vi "NewPeriodic Tasks.vi"(8 "error in":errorcluster) -> ()   [LabVIEW 2017]
doc: "This VI runs in parallel to other tasks. It can contain as many user-defined periodic loops as you need. These can carry out PID or other sorts of timed response."
uses:
  <vilib>/Analysis/baseanly.llb/Mean (DBL).vi
  <vilib>/Rock Robotics/WPI/Utilities/WPI_GetSetVariantRefNum.vi
  Robot Global Data.vi
  <vilib>/Rock Robotics/Network Tables/NT Write Number.vi
  <vilib>/Rock Robotics/Network Tables/NT Write Numeric Array.vi
  <vilib>/Analysis/NI_AALBase.lvlib
panel:
  out "Arrayval":dbl
  out "Accelerations":T1
  out "Joy Y":dbl(graph)
  out "Avg Y":dbl
  out "Mean":dbl(graph)
  out "Current Joy Y Value":dbl
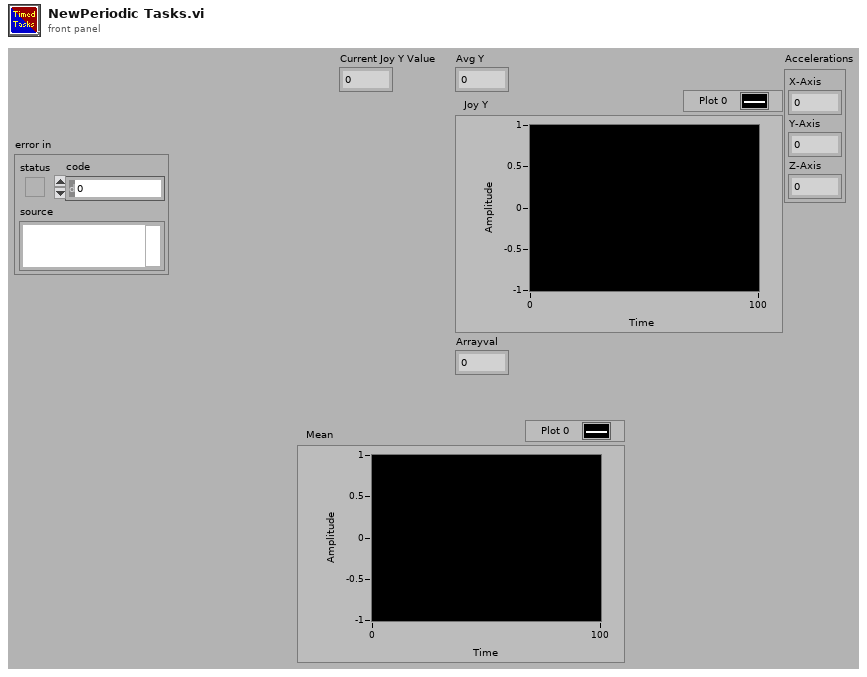
[diagram p1: front panel]
types:
  T1 = cluster{"X-Axis":dbl, "Y-Axis":dbl, "Z-Axis":dbl}
  T2 = typedef "WPI_JoystickDevRef.ctl" = cluster{"Device":T3}
  T3 = typedef "WPI_JoystickDeviceEnum.ctl" = enum16{"USB 0", "USB 1", "USB 2", "USB 3", "USB 4", "USB 5"}
  T4 = typedef "WPI_RobotDriveDevRef.ctl" = cluster{"DevStatus":errorcluster, "Motors[]":T5[], "Square Inputs":bool, "Max Output":dbl}
  T5 = typedef "WPI_MotorControlDeviceRef.ctl" = cluster{"DeviceStatus":errorcluster, "Type":T6, "PWM":cluster{"PWM Channel":T7, "DeadBand":T8}, "CAN":cluster{"Device Number":u8, "SetOutput VI Ref":variant, "GetOutput VI Ref":variant, "Enable VI Ref":variant, "Disable VI Ref":variant, "Data":variant}, "Invert":bool, "DIO PWM":cluster{"PWM \"Enable\" Channel":T7, "DIOChannel":T9, "PWM Rate":dbl}}
  T6 = typedef "WPI_MotorControlType.ctl" = enum16{"PWM", "CAN", "DIO PWM"}
  T7 = typedef "FPGA_DIOPWMChannel.ctl" = enum8{"PWM 0", "PWM 1", "PWM 2", "PWM 3", "PWM 4", "PWM 5", "PWM 6", "PWM 7", "PWM 8", "PWM 9", "PWM MXP 0", "PWM MXP 1", "PWM MXP 2", "PWM MXP 3", "PWM MXP 4", "PWM MXP 5", "PWM MXP 6", "PWM MXP 7", "PWM MXP 8", "PWM MXP 9", "Invalid"}
  T8 = typedef "WPI_PWMDeadband.ctl" = cluster{"Name":string, "maxPositivePwm":i32, "minPositivePwm":i32, "centerPwm":i32, "maxNegativePwm":i32, "minNegativePwm":i32, "angularRange":u16}
  T9 = typedef "FPGA_DIOChannel.ctl" = enum8{"DIO 0", "DIO 1", "DIO 2", "DIO 3", "DIO 4", "DIO 5", "DIO 6", "DIO 7", "DIO 8", "DIO 9", "DIO MXP 0", "DIO MXP 1", "DIO MXP 2", "DIO MXP 3", "DIO MXP 4", "DIO MXP 5", "DIO MXP 6", "DIO MXP 7", "DIO MXP 8", "DIO MXP 9", "DIO MXP 10", "DIO MXP 11", "DIO MXP 12", "DIO MXP 13", "DIO MXP 14", "DIO MXP 15", "SPI Port CS1", "SPI Port CS2", "SPI Port CS3", "SPI Port MISO", "SPI Port MOSI", "Invalid"}
  T10 = typedef "WPI_AccelerometerDevRef.ctl" = cluster{"DevStatus":errorcluster, "Scaling":T11, "Analog Channels":T12, "I2C Bus":T14, "SPI Bus":T15, "Accel Range":T16, "ADXL Axes":T17, "Handle":i32, "Device Address":u8, "Accel Type":enum16{"Analog", "ADXL345 I2C", "ADXL345 SPI", "Internal", "ADXL362 SPI"}}
  T11 = typedef "WPI_AccelerometerScaling.ctl" = cluster{"Gain (VoltsPerG)":dbl, "Center Voltage":dbl}
  T12 = typedef "WPI_AccelerometerAnalogChannels.ctl" = cluster{"X-Axis":T13, "Y-Axis":T13, "Z-Axis":T13}
  T13 = typedef "FPGA_AIChannel.ctl" = enum8{"AI 0", "AI 1", "AI 2", "AI 3", "AI MXP 0", "AI MXP 1", "AI MXP 2", "AI MXP 3", "Invalid"}
  T14 = typedef "i2c_bus.ctl" = enum16{"I2C On-Board", "I2C MXP", "Invalid"}
  T15 = typedef "spi_bus.ctl" = enum16{"SPI On-Board, CS0", "SPI On-Board, CS1", "SPI On-Board, CS2", "SPI On-Board, CS3", "SPI MXP", "Invalid"}
  T16 = typedef "ADXL345 Range.ctl" = u8
  T17 = typedef "WPI_AccelerometerADXL345 Axes.ctl" = cluster{"X-Axis":bool, "Y-Axis":bool, "Z-Axis":bool}
  T18 = typedef "WPI_GyroDevRef.ctl" = cluster{"DevStatus":errorcluster, "Analog Channel":T13, "Gain (VoltsPerDegree/Second)":dbl, "Gyro Type":enum16{"Analog", "XRS450"}, "Handle":i32, "SPI Bus":T15, "Device Found":bool, "Sample Rate":dbl, "Calibrate On Open":bool, "Offset":dbl}
  T19 = cluster{"JoystickDevRef":T2, "RobotDriveDevRef":T4}
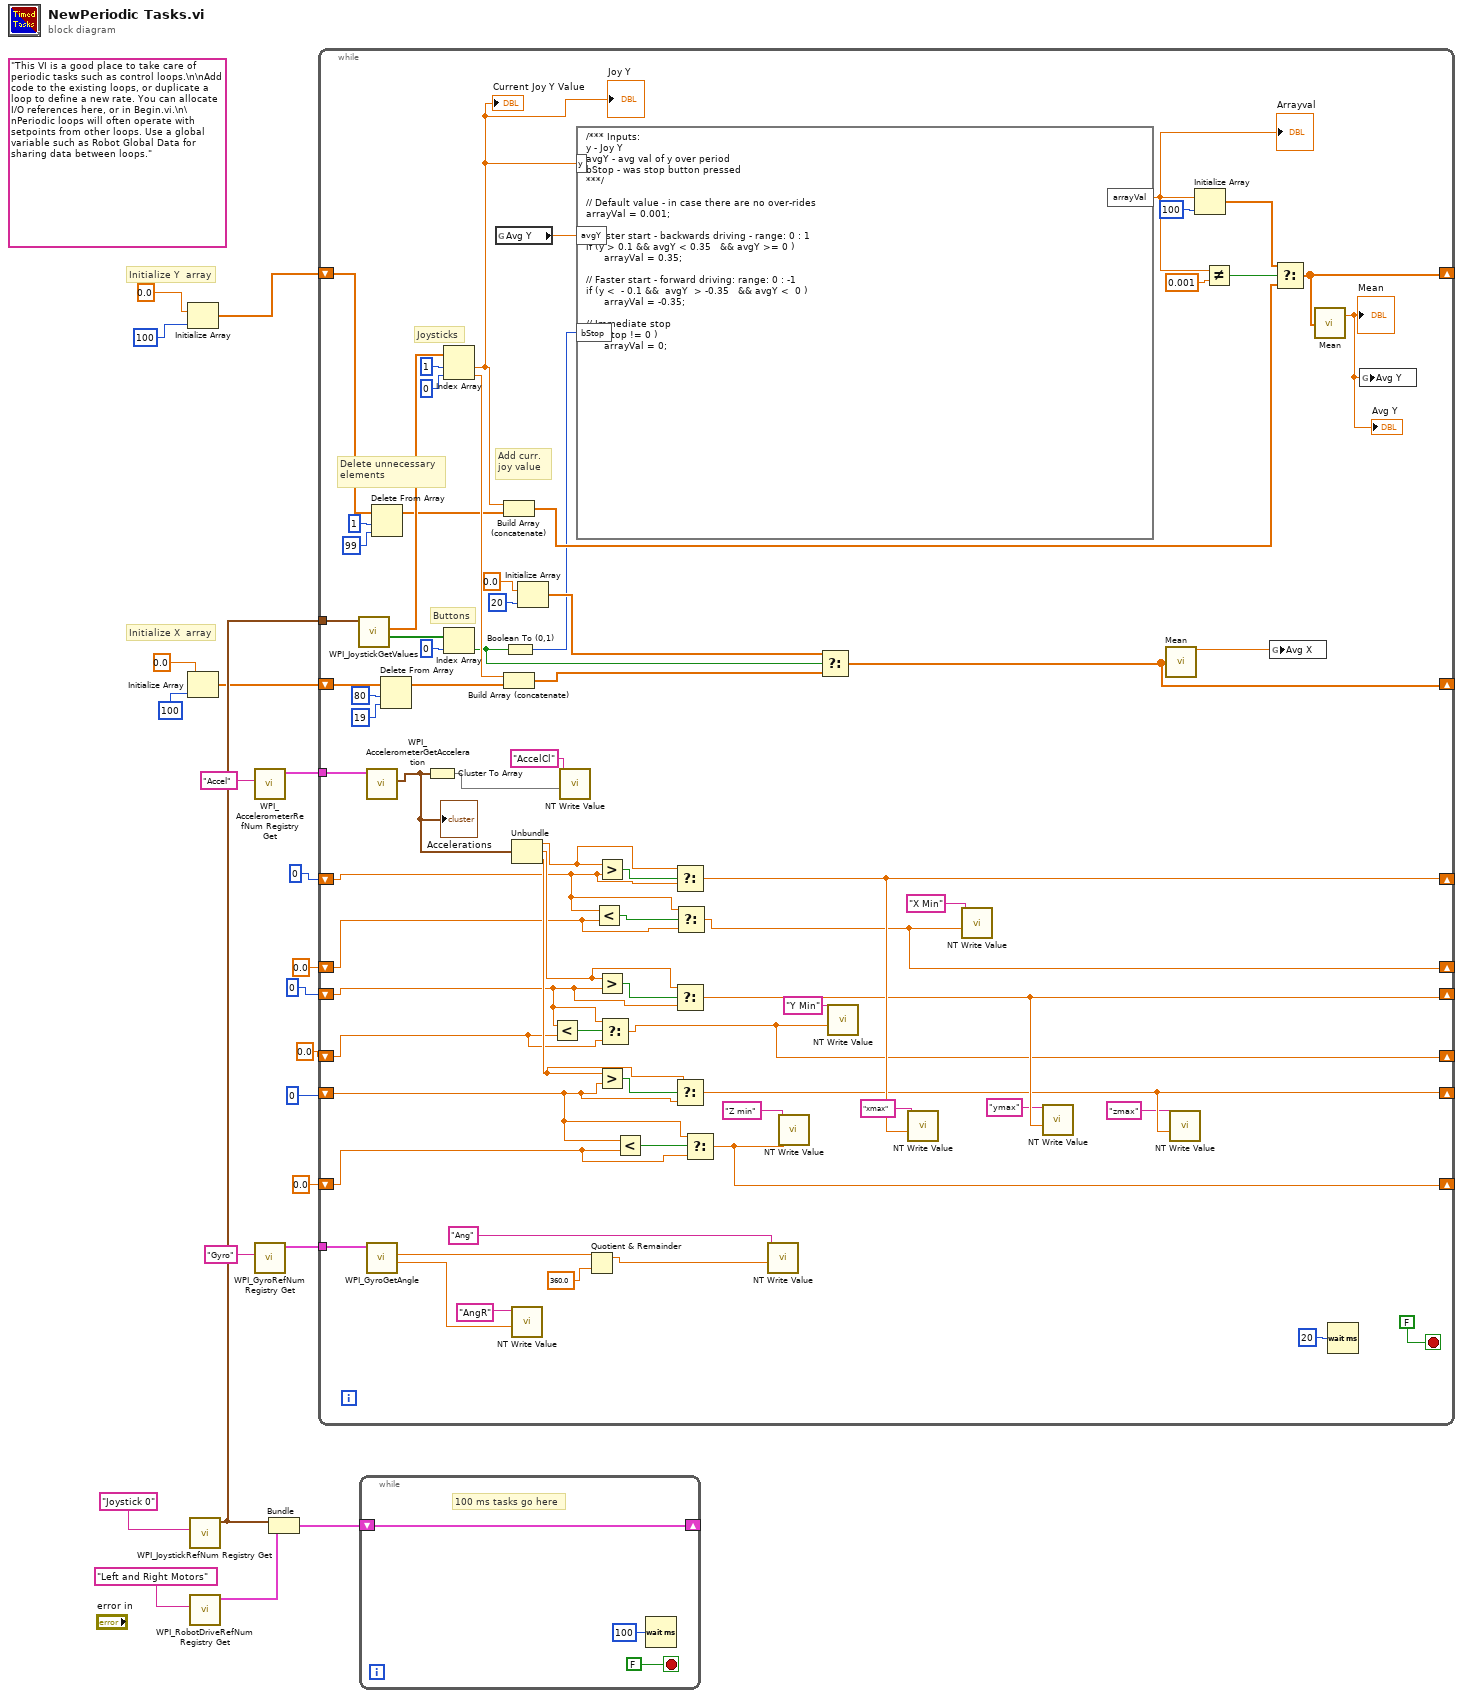
[diagram p0: block diagram]
diagram:
  (unwired) "This VI is a good place to take care of periodic tasks such as control loops.\n\nAdd code to the existing loops, or duplicate a loop to define a new rate. You can allocate I/O references here, or in Begin.vi.\n\nPeriodic loops will often operate with setpoints from other loops. Use a global variable such as Robot Global Data for sharing data between loops."
  # "Initialize X  array"
  # "Initialize Y  array"
  n1 = Initialize Array(0.0 ("element"), 100 ("dimension size")) -> (w14:dbl[])
  n2 = Initialize Array(0.0 ("element"), 100 ("dimension size")) -> (w13:dbl[])
  n3 = call <vilib>:"WPI_JoystickRefNum Registry Get.vi"("refnum name"="Joystick 0") -> ("JoystickDevRef"=w17:T2)  [unwired: 1 in, 9 out]
  n4 = call <vilib>:"WPI_RobotDriveRefNum Registry Get.vi"("refnum name"="Left and Right Motors") -> ("RobotDriveDevRef"=w19:T4)  [unwired: 1 in, 9 out]
  n5 = call <vilib>:"WPI_AccelerometerRefNum Registry Get.vi"("refnum name"="Accel") -> ("AccelerometerDevRef"=w9:T10)  [unwired: 9 in, 1 out]
  n6 = call <vilib>:"WPI_GyroRefNum Registry Get.vi"("refnum name"="Gyro") -> ("GyroDevRef"=w7:T18)  [unwired: 9 in, 1 out]
  n7 = Bundle("JoystickDevRef"=w17, "RobotDriveDevRef"=w19) -> (w18:T19)  [unwired: 1 out]
  n8 = while {
    tunnel: w17 -> [w92]
    shift-right: [w66] -> _
    shift-left: w14 -> [w89]
    shift-right: [w85] -> _
    shift-left: w13 -> [w79]
    tunnel: w9 -> [w61]
    tunnel: w7 -> [w60]
    shift-right: [w44] -> _
    shift-left: 0 -> [w35]
    shift-right: [w43] -> _
    shift-left: 0 -> [w30]
    shift-right: [w42] -> _
    shift-left: 0 -> [w26]
    shift-right: [w33] -> _
    shift-left: 0.0 ("X-Axis") -> [w32]
    shift-right: [w28] -> _
    shift-left: 0.0 ("Y-Axis") -> [w27]
    shift-right: [w23] -> _
    shift-left: 0.0 ("Z-Axis") -> [w22]
    stop <- FALSE stop-if-true
    # "Add curr. \njoy value"
    # "Delete unnecessary \nelements"
    # "Joysticks"
    # "Buttons"
    n9 = call <vilib>:"WPI_JoystickGetValues.vi"("JoystickDevRef"=w92) -> ("Buttons"=w88:bool[], "Axes"=w91:dbl[])  [unwired: 6 in, 3 out]
    n10 = call <vilib>:"WPI_AccelerometerGetAcceleration.vi"("AccelerometerDevRef"=w61) -> ("Accelerations"=w51:T1)  [unwired: 8 in, 2 out]
    "Accelerations" <- w51
    n11 = call <vilib>:"WPI_GyroGetAngle.vi"("GyroDevRef"=w60) -> ("Angular Rate"=w58:dbl, "Angle"=w53:dbl)  [unwired: 7 in, 2 out]
    n12 = Delete From Array(array=w89, length=1, index=99) -> (array with subset deleted=w71:dbl[])  [unwired: 1 out]
    n13 = Delete From Array(array=w79, length=80, index=19) -> (array with subset deleted=w81:dbl[])  [unwired: 1 out]
    n14 = Cluster To Array(cluster=w51) -> (array=w59:dbl[])
    n15 = Index Array(array=w91, index #1=1 ("index"), index #2=0 ("index")) -> (element #1=w62:dbl, element #2=w77:dbl)
    "Current Joy Y Value" <- w62
    "Joy Y" <- w62
    n16 = Index Array(array=w88, index=0) -> (element=w67:bool)
    n17 = global read "Robot Global Data.vi" "Avg Y"() -> (w69:dbl)
    n18 = Build Array (concatenate)(w62, w71) -> (w70:dbl[])
    n19 = Build Array (concatenate)(w77, w81) -> (w78:dbl[])
    n20 = Boolean To (0,1)(Boolean=w67) -> (0, 1=w68:i16)
    n21 = Unbundle(w51) -> ("X-Axis"=w49:dbl, "Y-Axis"=w46:dbl, "Z-Axis"=w45:dbl)
    n22 = call-poly <vilib>:"NT Write Value.vi"("Numeric"=w58, "Name"="AngR") -> ()  [unwired: 9 in, 1 out]
    n23 = Initialize Array(0.0 ("element"), 20 ("dimension size")) -> (w84:dbl[])
    n24 = Less?(x=w30, y=w27) -> (x < y?=w31:bool)
    n25 = call-poly <vilib>:"NT Write Value.vi"("Numeric Array"=w59, "Name"="AccelCl") -> ()  [unwired: 9 in, 1 out]
    n26 = formula code="/*** Inputs:\ny - Joy Y\navgY - avg val of y over period\nbStop - was stop button pressed\n***/\n\n// Default value - in case there are no over-rides\narrayVal = 0.001;\n\n// Faster start - backwards driving - range: 0 : 1\nif (y > 0.1 && avgY < 0.35   && avgY >= 0 )\n      arrayVal = 0.35;\n\n// Faster start - forward driving: range: 0 : -1\nif (y <  - 0.1 &&  avgY  > -0.35   && avgY <  0 )\n      arrayVal = -0.35;\n\n// Immediate stop\nif (bStop != 0 )\n      arrayVal = 0;"("y"=w62, "avgY"=w69, "bStop"=w68) -> ("arrayVal"=w63:dbl)
    "Arrayval" <- w63
    n27 = Quotient & Remainder(x=w53, y=360.0) -> (x-y*floor(x/y)=w52:dbl)  [unwired: 1 out]
    n28 = Less?(x=w35, y=w32) -> (x < y?=w36:bool)
    n29 = Greater?(x=w49, y=w35) -> (0:w50:bool)
    n30 = Greater?(x=w46, y=w30) -> (0:w48:bool)
    n31 = Greater?(x=w45, y=w26) -> (0:w47:bool)
    n32 = Select(t=w30, s=w31, f=w27) -> (s? t:f=w28:dbl)
    n33 = Less?(x=w26, y=w22) -> (x < y?=w24:bool)
    n34 = Select(t=w49, s=w50, f=w35) -> (s? t:f=w44:dbl)
    n35 = Select(t=w46, s=w48, f=w30) -> (s? t:f=w43:dbl)
    n36 = Select(t=w45, s=w47, f=w26) -> (s? t:f=w42:dbl)
    n37 = Select(t=w35, s=w36, f=w32) -> (s? t:f=w33:dbl)
    n38 = Select(t=w26, s=w24, f=w22) -> (s? t:f=w23:dbl)
    n39 = call-poly <vilib>:"NT Write Value.vi"("Numeric"=w52, "Name"="Ang") -> ()  [unwired: 9 in, 1 out]
    n40 = call-poly <vilib>:"NT Write Value.vi"("Numeric"=w23, "Name"="Z min") -> ()  [unwired: 9 in, 1 out]
    n41 = Select(t=w84, s=w67, f=w78) -> (s? t:f=w85:dbl[])
    n42 = call-poly <vilib>:"NT Write Value.vi"("Numeric"=w28, "Name"="Y Min") -> ()  [unwired: 9 in, 1 out]
    n43 = call-poly <vilib>:"NT Write Value.vi"("Numeric"=w44, "Name"="xmax") -> ()  [unwired: 9 in, 1 out]
    n44 = call-poly <vilib>:"NT Write Value.vi"("Numeric"=w33, "Name"="X Min") -> ()  [unwired: 9 in, 1 out]
    n45 = call-poly <vilib>:"NT Write Value.vi"("Numeric"=w43, "Name"="ymax") -> ()  [unwired: 9 in, 1 out]
    n46 = call-poly <vilib>:"Mean.vi"("X"=w85) -> ("mean"=w38:dbl)  [unwired: 1 out]
    n47 = call-poly <vilib>:"NT Write Value.vi"("Numeric"=w42, "Name"="zmax") -> ()  [unwired: 9 in, 1 out]
    n48 = Initialize Array(w63, 100 ("dimension size")) -> (w73:dbl[])
    n49 = Not Equal?(x=w63, y=0.001) -> (x != y?=w65:bool)
    n50 = global write "Robot Global Data.vi" "Avg X"(w38) -> ()
    n51 = Select(t=w73, s=w65, f=w70) -> (s? t:f=w66:dbl[])
    n52 = call-poly <vilib>:"Mean.vi"("X"=w66) -> ("mean"=w37:dbl)  [unwired: 1 out]
    "Mean" <- w37
    "Avg Y" <- w37
    n53 = Wait (ms)(milliseconds to wait=u32 20) -> ()  [unwired: 1 out]
    n54 = global write "Robot Global Data.vi" "Avg Y"(w37) -> ()
  }
  n55 = while {
    shift-right: [w95] -> _
    shift-left: w18 -> [w95]
    stop <- FALSE stop-if-true
    # "100 ms tasks go here"
    n56 = Wait (ms)(milliseconds to wait=u32 100) -> ()  [unwired: 1 out]
  }
